vi "CA Voltage Check.vi"(6 "Digitizer Settings":T1={"Digitizer delay (us) "=0.0, "rf points per line"=2048, "lines per plane"=128, "Samp Rate (Hz)"=100000000.0, "Additional dig delay (us)"=0.0, "Voltage Scale"=0.4, "Pre-Looks"=0, "Offset delay (us)"=0.0, "bits A/D"=8, "Avg Num"=1, "DigTimeOut"=5.0, "Rel Dig Delay"=0.0, "Dig Ch"=0, "LeCroyCluster"={"LeCroy Channels"=[TRUE, FALSE, FALSE, FALSE], "LC read pt offset"=0.0, "Sweep Avg"=FALSE}, "Main Digitizer"=enum."NI Digitizer", "Dig Config"=enum."Single channel", "Digitizer ID Cluster"={"Acqiris/Alazar/SP ID"=[], "NI Instr Handles"=[], "LeCroy VISA"="", "GaGe Handle"={"Handle"=0, "Sample size"=0, "Resolution"=0, "Offset"=0, "Channels"=0, "Boards"=0}, "ATS Ref"="ATS9350", "Acqiris Address"=["PCI::INSTR0"], "ADQRef"=refnum, "adq_cu_ptr"=refnum}, "Trigger Settings"={"Trig Source"=1, "Trig Coupling"=0, "Trig Slope"=0, "Level (mV)"=1500.0}, "Bulk Acq"=FALSE, "Bulk Start Indexes"=[], "Data Ref RF"=refnum, "NI ID/Channel"=[], "Total Dig CH"=1, "Xtra Ann Trig delay (us)"=10.0, "Fix Z Delay?"=FALSE, "One Way Transmission?"=FALSE, "Data Ref Log"=refnum} {"Trigger Settings"."Trig Slope" items=["Positive", "Negative"]; "Trigger Settings"."Level (mV)" format="%.2f"; "Trigger Settings"."Trig Coupling" items=["DC 1 MOhm", "AC 1 MOhm", "DC 50 Ohm", "AC 50 Ohm"]; "Trigger Settings"."Trig Source" items=["Chan 1", "External"]; "Rel Dig Delay" format="%.2f"; "DigTimeOut" format="%.2f"; "Avg Num" min=1; "Offset delay (us)" format="%.2f"; "Additional dig delay (us)" format="%.2f"; "Digitizer delay (us)" format="%.2f"}, 8 "Up Once?":bool, 9 "All Peak in":i32[](array[numeric]), 10 "count in":i32, 11 "valid peak in":i32[](array[numeric])) -> (0 "Up Once Out":bool, 1 "All Peak Out":i32[](array[numeric]), 2 "count out":i32, 3 "valid peak out":i32[](array[numeric]), 4 "low %":dbl, 5 "clip%":dbl)   [LabVIEW 2022 SP3]
uses:
  DigitizerSettings.ctl
  Digitizer.ctl
  DigConfig.ctl
  DigitizerID.ctl
  C:/Windows/System32/ADQAPI_dotNet_helper.dll
  <vilib>/Analysis/NI_AALPro.lvlib
panel:
  in  "clip Frac Thresh":dbl=0.05
  in  "Low Frac Thresh":dbl=0.95
  # "Step up voltage if over \"clip Frac Thresh\"  of valid events are saturated"
  # "Step down voltage  if \"Low Frac Thresh\" % of events are just using 7 bits. Account for nonuniform voltage jumps"
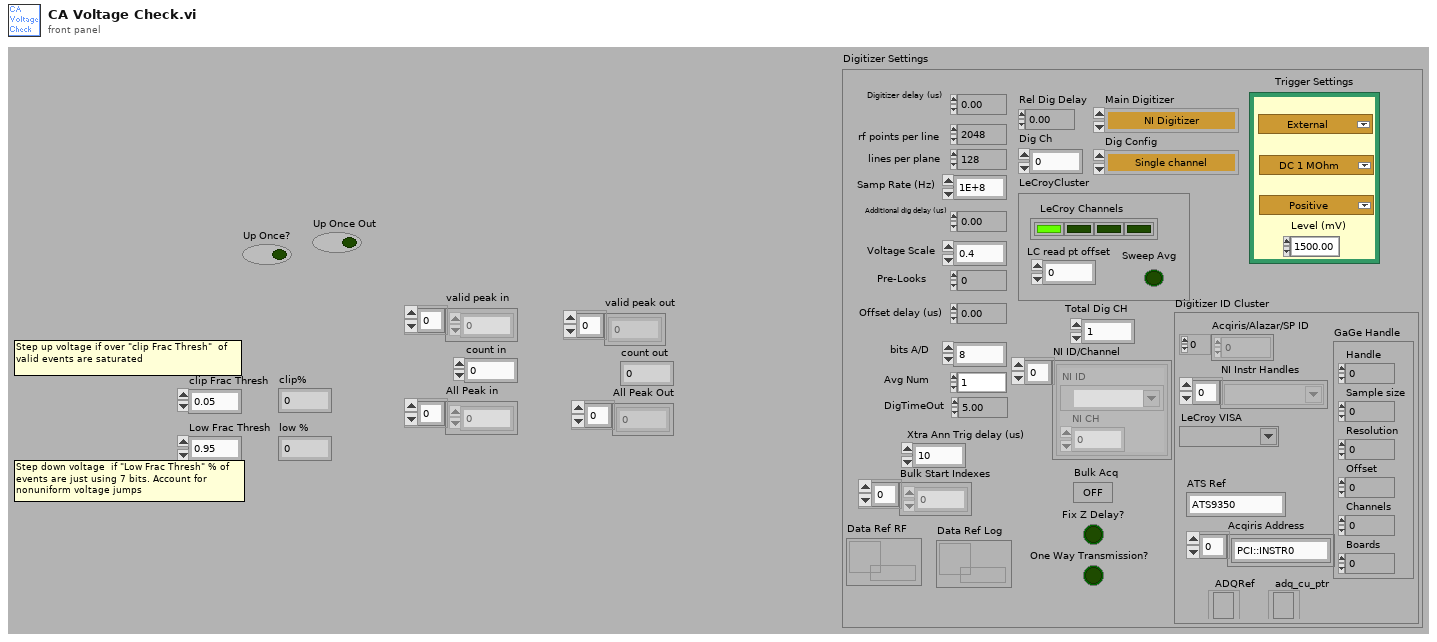
[diagram p1: front panel]
types:
  T1 = typedef "DigitizerSettings.ctl" = cluster{"Digitizer delay (us) ":dbl, "rf points per line":i32, "lines per plane":i32, "Samp Rate (Hz)":dbl, "Additional dig delay (us)":dbl, "Voltage Scale":dbl, "Pre-Looks":i32, "Offset delay (us)":dbl, "bits A/D":i8, "Avg Num":i32, "DigTimeOut":sgl, "Rel Dig Delay":sgl, "Dig Ch":i32, "LeCroyCluster":cluster{"LeCroy Channels":bool[], "LC read pt offset":dbl, "Sweep Avg":bool}, "Main Digitizer":T2, "Dig Config":T3, "Digitizer ID Cluster":T4, "Trigger Settings":cluster{"Trig Source":u16, "Trig Coupling":u16, "Trig Slope":u16, "Level (mV)":dbl}, "Bulk Acq":bool, "Bulk Start Indexes":i32[], "Data Ref RF":refnum<data-value>, "NI ID/Channel":cluster{"NI ID":refnum<k15>, "NI CH":i32}[], "Total Dig CH":i32, "Xtra Ann Trig delay (us)":dbl, "Fix Z Delay?":bool, "One Way Transmission?":bool, "Data Ref Log":refnum<data-value>}
  T2 = typedef "Digitizer.ctl" = enum16{"Acqiris Digitizer", "NI Digitizer", "LeCroy", "GaGe", "AlazarTech", "No Digitizer", "Teledyne"}
  T3 = typedef "DigConfig.ctl" = enum16{"Single channel", "2 Chans w/ 2 Acqiris", "2 Chans w/ 1 Acqiris", "5-CH Pulser New", "5-CH pulser w/ ann array", "5-pass style ann array", "Empty"}
  T4 = typedef "DigitizerID.ctl" = cluster{"Acqiris/Alazar/SP ID":u32[], "NI Instr Handles":refnum<k15>[], "LeCroy VISA":refnum<visa-resource-name>, "GaGe Handle":cluster{"Handle":u32, "Sample size":u32, "Resolution":i32, "Offset":i32, "Channels":u32, "Boards":u32}, "ATS Ref":string, "Acqiris Address":string[], "ADQRef":refnum<k24>, "adq_cu_ptr":refnum<k24>}
  T5 = cluster{"lower":dbl, "upper":dbl, "inclusion":enum32{"lower", "upper", "both", "neither"}}[]
  T6 = cluster{"Voltage Scale":i16, "Offset":dbl, "Coupling":u16}
  T7 = cluster{"Voltage Scale":dbl, "Offset":dbl, "Coupling":u16}
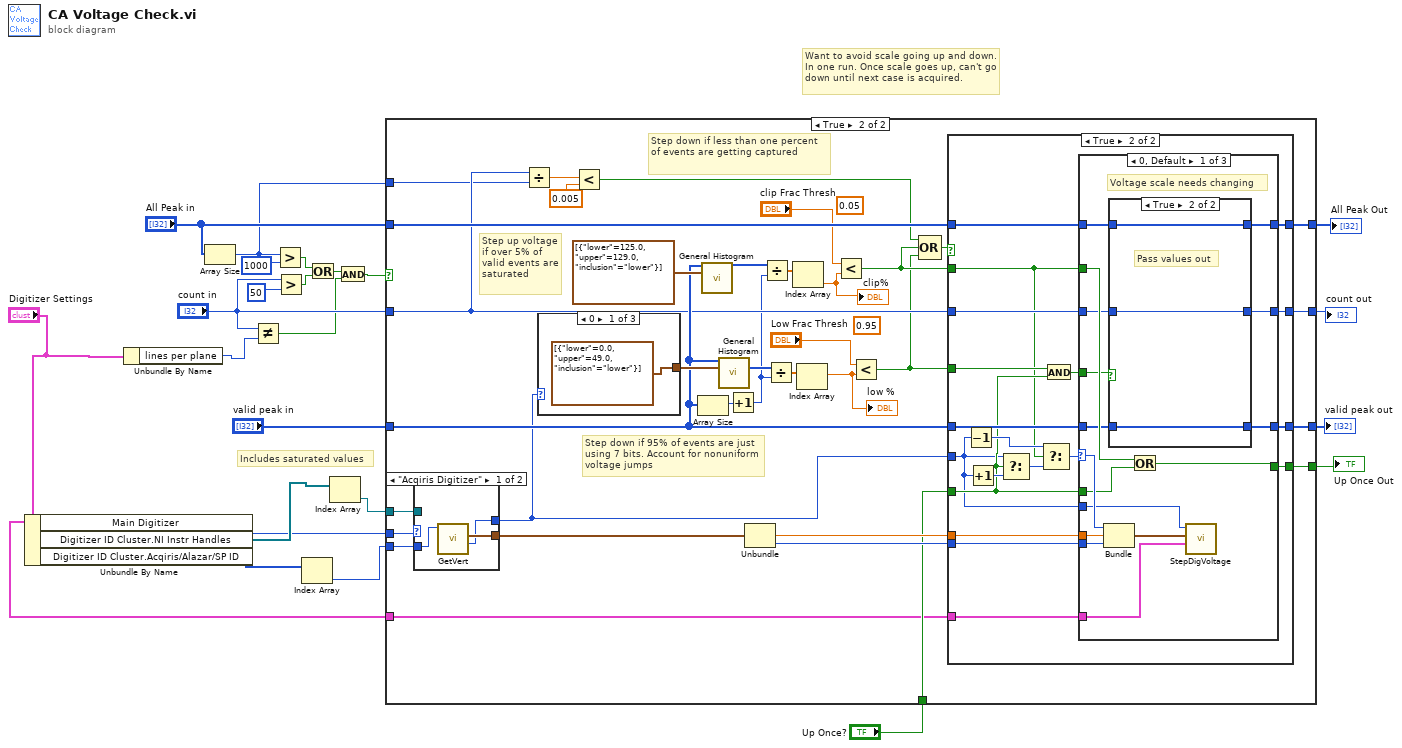
[diagram p0: block diagram]
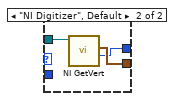
[diagram p3: hidden frame]
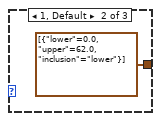
[diagram p4: hidden frame]
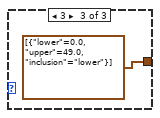
[diagram p5: hidden frame]
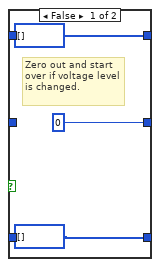
[diagram p7: hidden frame]
diagram:
  # "Want to avoid scale going up and down. In one run. Once scale goes up, can't go down until next case is acquired."
  # "Includes saturated values"
  n1 = Unbundle By Name("Digitizer Settings") -> ("Main Digitizer"=w1:T2, "Digitizer ID Cluster.NI Instr Handles"=w4:refnum<k15>[], "Digitizer ID Cluster.Acqiris/Alazar/SP ID"=w6:u32[])
  n2 = Unbundle By Name("Digitizer Settings") -> ("lines per plane"=w3:i32)
  n3 = Array Size(array="All Peak in") -> (size(s)=w14:i32)
  n4 = Not Equal?(x="count in", y=w3) -> (x != y?=w8:bool)
  n5 = Greater?(x=w14, y=1000) -> (0:w15:bool)
  n6 = Greater?(x="count in", y=50) -> (0:w16:bool)
  n7 = Index Array(array=w6) -> (element=w5:u32)  [unwired: 1 in]
  n8 = Or(x=w15, y=w16) -> (x .or. y?=w10:bool)
  n9 = Index Array(array=w4) -> (element=w7:refnum<k15>)  [unwired: 1 in]
  n10 = And(x=w10, y=w8) -> (x .and. y?=w9:bool)
  n11 = case shown="True" w9 {
    tunnel: "All Peak in" -> [w26 w48]
    tunnel: "count in" -> [w27 w45]
    tunnel: [w27 w52] -> w22
    tunnel: [w26 w54] -> w21
    tunnel: "valid peak in" -> [w25 w46]
    tunnel: [w25 w53] -> w19
    tunnel: w14 -> [_ w44]
    tunnel: "Up Once?" -> [w24 w38]
    tunnel: [w24 w37] -> w12
    tunnel: w1 -> [_ w32]
    tunnel: w5 -> [_ w31]
    tunnel: w7 -> [_ w30]
    tunnel: "Digitizer Settings" -> [_ w28]
    frame False {
    }
    frame True {
      (unwired) 0.05
      (unwired) 0.95
      # "Step down if less than one percent of events are getting captured"
      # "Step down if 95% of events are just using 7 bits. Account for nonuniform voltage jumps"
      # "Step up voltage if over 5% of valid events are saturated"
      n12 = case shown="\"Acqiris Digitizer\"" w32 {
        tunnel: [w65 w68] -> w33
        tunnel: w31 -> [w64 _]
        tunnel: w30 -> [_ w67]
        tunnel: [w63 w66] -> w29
        frame "Acqiris Digitizer" {
          n13 = call "GetVert.vi"("InstrumentID"=w64) -> ("index of element"=w63:i32, "V scale"=w65:T6)  [unwired: 3 in, 2 out]
        }
        frame "NI Digitizer", Default {
          n14 = call "NI GetVert.vi"("InstrumentID"=w67) -> ("index of element"=w66:i32, "V scale"=w68:T7)  [unwired: 2 in, 3 out]
        }
      }
      n15 = Divide(x=w45, y=w44) -> (x/y=w43:dbl)
      n16 = case shown="0" w29 {
        tunnel: [T5 [{"lower"=0.0, "upper"=49.0, "inclusion"=enum."lower"}] ("Bins") T5 [{"lower"=0.0, "upper"=62.0, "inclusion"=enum."lower"}] ("Bins") T5 [{"lower"=0.0, "upper"=49.0, "inclusion"=enum."lower"}] ("Bins")] -> w59
        frame 0 {
        }
        frame 1, Default {
        }
        frame 3 {
        }
      }
      n17 = Less?(x=w43, y=0.005) -> (x < y?=w41:bool)
      n18 = Array Size(array=w46) -> (size(s)=w47:i32)
      n19 = call <vilib>:"General Histogram.vi"("X"=w46, "Bins"=T5 [{"lower"=125.0, "upper"=129.0, "inclusion"=enum."lower"}]) -> ("Histogram"=w61:i32[])  [unwired: 4 in, 9 out]
      n20 = call <vilib>:"General Histogram.vi"("X"=w46, "Bins"=w59) -> ("Histogram"=w58:i32[])  [unwired: 4 in, 9 out]
      n21 = Increment(x=w47) -> (x+1=w40:i32)
      n22 = Unbundle(w33) -> ("Offset"=w50:dbl, "Coupling"=w51:u16)  [unwired: 1 out]
      n23 = Divide(x=w61, y=w40) -> (x/y=w60:dbl[])
      n24 = Divide(x=w58, y=w40) -> (x/y=w57:dbl[])
      n25 = Index Array(array=w60) -> (element=w56:dbl)  [unwired: 1 in]
      "clip%" <- w56
      n26 = Index Array(array=w57) -> (element=w55:dbl)  [unwired: 1 in]
      "low %" <- w55
      n27 = Less?(x="clip Frac Thresh", y=w56) -> (x < y?=w39:bool)
      n28 = Less?(x="Low Frac Thresh", y=w55) -> (x < y?=w36:bool)
      n29 = Compound Arithmetic op=OR(w41, w39, w36) -> (w49:bool)
      n30 = case shown="True" w49 {
        tunnel: [w75 w94] -> w54
        tunnel: w48 -> [w75 w87]
        tunnel: [w73 w92] -> w53
        tunnel: [w74 w93] -> w52
        tunnel: w45 -> [w74 w85]
        tunnel: w51 -> [_ w91]
        tunnel: w50 -> [_ w90]
        tunnel: w29 -> [_ w77]
        tunnel: w39 -> [_ w78]
        tunnel: w46 -> [w73 w86]
        tunnel: w38 -> [w72 w81]
        tunnel: [w72 w82] -> w37
        tunnel: w36 -> [_ w79]
        tunnel: w28 -> [_ w76]
        frame False {
          # "Normal voltage range decision and vlaues are passed along"
        }
        frame True {
          n31 = Decrement(x=w77) -> (x-1=w89:i32)
          n32 = Increment(x=w77) -> (x+1=w84:i32)
          n33 = Select(t=w77, s=w81, f=w84) -> (s? t:f=w83:i32)
          n34 = Select(t=w89, s=w78, f=w83) -> (s? t:f=w88:i32)
          n35 = And(x=w79, y=w81) -> (x .and. y?=w80:bool)
          n36 = case shown="0, Default" w88 {
            selector: w88 -> [w105 _ _]
            tunnel: [w110 w120 w124] -> w94
            tunnel: [w109 w119 w123] -> w93
            tunnel: [w108 w118 w122] -> w92
            tunnel: w91 -> [w107 _ _]
            tunnel: w90 -> [w106 _ _]
            tunnel: w87 -> [w100 w120 w124]
            tunnel: w85 -> [w99 w119 w123]
            tunnel: w86 -> [w98 w118 w122]
            tunnel: w78 -> [w102 _ _]
            tunnel: [w103 w117 w121] -> w82
            tunnel: w81 -> [w101 w117 w121]
            tunnel: w80 -> [w97 _ _]
            tunnel: w77 -> [w96 _ _]
            tunnel: w76 -> [w95 _ _]
            frame 0, Default {
              # "Voltage scale needs changing"
              n37 = Bundle(w105, "Offset"=w106, "Coupling"=w107) -> (w104:cluster{i32, "Offset":dbl, "Coupling":u16})  [unwired: 1 out]
              n38 = case shown="True" w97 {
                tunnel: [i16[] [] ("All Peak in") w116] -> w110
                tunnel: [0 ("count in") w115] -> w109
                tunnel: [i16[] [] ("valid peak in") w114] -> w108
                tunnel: w100 -> [_ w116]
                tunnel: w99 -> [_ w115]
                tunnel: w98 -> [_ w114]
                frame False {
                  # "Zero out and start over if voltage level is changed."
                }
                frame True {
                  # "Pass values out"
                }
              }
              n39 = Or(x=w102, y=w101) -> (x .or. y?=w103:bool)
              n40 = call "StepDigVoltage.vi"("Digitizer Settings"=w95, "Voltage Settings"=w104, "Prev Vol Val"=w96) -> ()  [unwired: 2 in]
            }
            frame 7 {
              # "Pass values on. 7  means voltage high and larger voltage scale would be used if one were avaible."
            }
            frame -1 {
              # "Pass values on. -1 means voltage is low and a smaller  voltage scale would be used if one were avaible."
            }
          }
        }
      }
    }
  }
  "count out" <- w22
  "All Peak Out" <- w21
  "valid peak out" <- w19
  "Up Once Out" <- w12
